vi "Izvlechenie_kvadratnogo_kornya.vi"() -> ()   [LabVIEW 2018]
panel:
  out "Квадратный корень числа":dbl
  in  "Число":dbl
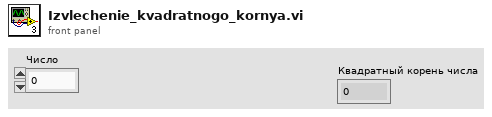
[diagram p1: front panel]
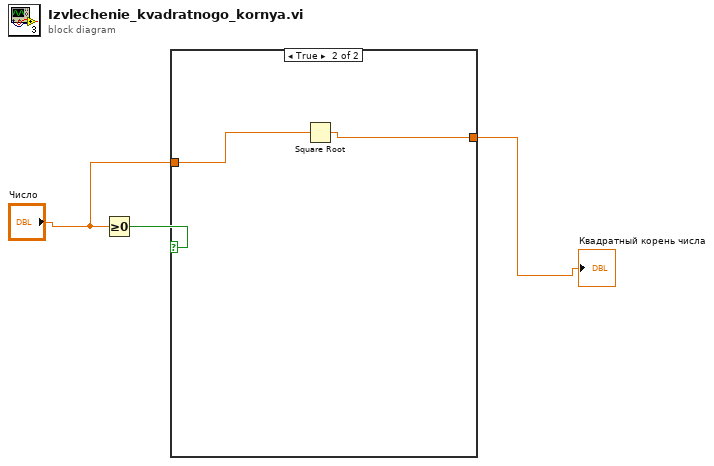
[diagram p0: block diagram]
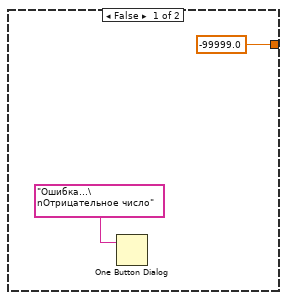
[diagram p2: hidden frame]
diagram:
  n1 = Greater Or Equal To 0?(x="Число") -> (x >= 0?=w3:bool)
  n2 = case shown="True" w3 {
    tunnel: "Число" -> [_ w7]
    tunnel: [-99999.0 w6] -> w1
    frame False {
      n3 = One Button Dialog(message="Ошибка...\nОтрицательное число") -> ()  [unwired: 1 in, 1 out]
    }
    frame True {
      n4 = Square Root(x=w7) -> (sqrt(x)=w6:dbl)
    }
  }
  "Квадратный корень числа" <- w1
